vi "Timer_Init.vi"(8 "error in (no error)":errorcluster) -> (0 "error out":errorcluster, 3 "Timer Data Reference (out)":refnum<data-value>)   [LabVIEW 2024]
doc: "Initialize the Timer DVR\n\n--------\nPaulo Rossi\nprossi@aurumautomation.ca\n©2024 Aurum Automation Inc.\nOpen-Sourced per GNU GPL v3\n\nYou should have received a copy of the GNU General Public License along with this program. If not, see <https://www.gnu.org/licenses/>."
uses:
  Timer_Data.ctl
panel:
  in  "Timer Data":T1 {"Cumulative Paused Time" format="%#_13g"; "Pause Elapsed Time" format="%#_13g"; "Pause Start Time" format="%#_13g"; "Target Time (s)" format="%#_13g"; "Time Elapsed (s)" format="%#_13g"; "Starting Time" format="%#_13g"}
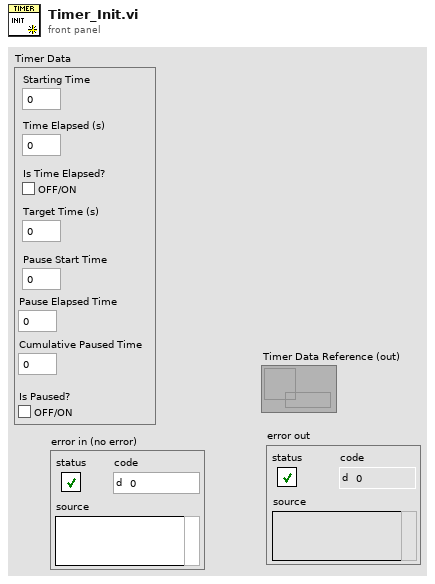
[diagram p1: front panel]
types:
  T1 = typedef "Timer_Data.ctl" = cluster{"Starting Time":dbl, "Time Elapsed (s)":dbl, "Is Time Elapsed?":bool, "Target Time (s)":dbl, "Pause Start Time":dbl, "Pause Elapsed Time":dbl, "Is Paused?":bool, "Cumulative Paused Time":dbl}
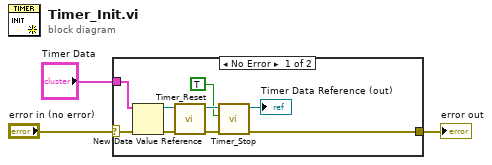
[diagram p0: block diagram]
diagram:
  n1 = case shown="No Error" "error in (no error)" {
    selector: "error in (no error)" -> [w11 w13]
    tunnel: [w5 w13] -> w2
    tunnel: "Timer Data" -> [w12 _]
    frame No Error {
      n2 = New Data Value Reference(data value=w12, error in=w11) -> (data value reference=w9:refnum<data-value>, error out=w10:errorcluster)
      n3 = call "Timer_Reset.vi"("error in (no error)"=w10, "Timer Data Reference (in)"=w9) -> ("error out"=w7:errorcluster, "Timer Data Reference (out)"=w8:refnum<data-value>)  [unwired: 8 in]
      n4 = call "Timer_Stop.vi"("error in (no error)"=w7, "Is Paused?"=TRUE, "Timer Data Reference (in)"=w8) -> ("error out"=w5:errorcluster, "Timer Data Reference (out)"=→"Timer Data Reference (out)":refnum<data-value>)  [unwired: 7 in]
    }
    frame Error {
    }
  }
  "error out" <- w2
